vi "Update FP and Show.vi"(8 "error in (no error)":errorcluster, 10 "Panel Ref":refnum<vi>, 11 "VI in":refnum<vi>) -> (0 "error out":errorcluster, 3 "VI out":refnum<vi>)   [LabVIEW 2021, in "Pop-Up.lvlib" / "Popup.lvclass"]
doc: "turn back on the front panel updates and show the FP on the screen - this should be done after all moving parts have been placed. this will be used for custom pop ups when the image size is unknown and the locations move.\n\n<b>Code Developed By:</b> +\nDaniel Coons +\nhttps://github.com/danielcoons/tsc-pop-up"
uses:
  Popup.lvclass
  Popup.lvclass/Popup.ctl
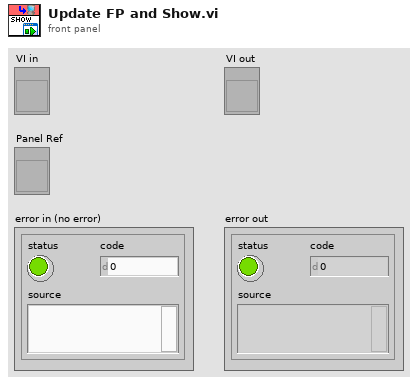
[diagram p1: front panel]
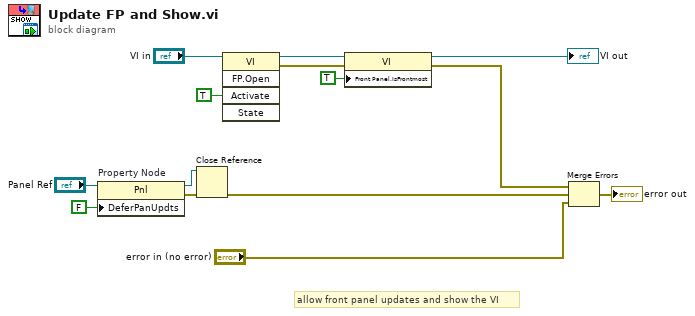
[diagram p0: block diagram]
diagram:
  # "allow front panel updates and show the VI"
  n1 = property on="Property Node" class="Pnl"(reference="Panel Ref", "DeferPanUpdts"=FALSE ("Defer Panel Updates")) -> (reference out=w9:refnum<vi>, error out=w10:errorcluster)  [unwired: 1 in]
  n2 = Close Reference(reference=w9, error in (no error)=w10) -> (error out=w6:errorcluster)
  n3 = invoke class="VI" method="FP.Open"(reference="VI in", "Activate"=TRUE ("Activate?")) -> (reference out=w3:refnum<vi>, error out=w5:errorcluster)  [unwired: 3 in, 3 out]
  n4 = property class="VI"(reference=w3, error in=w5, "Front Panel.IsFrontmost"=TRUE ("Front Panel Window:Is Frontmost")) -> (reference out=→"VI out":refnum<vi>, error out=w4:errorcluster)
  n5 = Merge Errors(w4, w6, "error in (no error)") -> (→"error out":errorcluster)
